vi "labels.get.vi"(8 "error in (no error)":errorcluster, 11 "labels in":refnum<class "labels.lvclass">) -> (0 "error out":errorcluster, 2 "labels":set{string}(c389), 3 "labels out":refnum<class "labels.lvclass">)   [LabVIEW 2020, in "nominal types.lvlib" / "labels.lvclass"]
uses:
  labels.lvclass
  labels.lvclass/labels.ctl
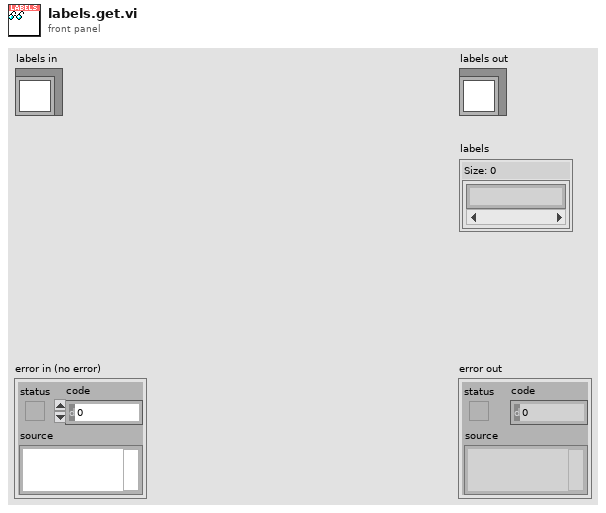
[diagram p1: front panel]
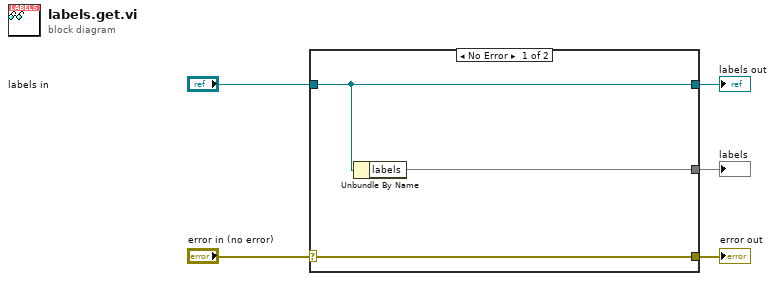
[diagram p0: block diagram]
diagram:
  n1 = case shown="No Error" "error in (no error)" {
    selector: "error in (no error)" -> [w8 w9]
    tunnel: [w8 w9] -> w4
    tunnel: [w7 w10] -> w2
    tunnel: "labels in" -> [w7 w10]
    tunnel: [w6 _] -> w1
    frame No Error {
      n2 = Unbundle By Name(w7) -> ("labels"=w6:set{string})
    }
    frame Error {
    }
  }
  "error out" <- w4
  "labels out" <- w2
  "labels" <- w1
